vi "Measure_Main.vi"(0 "time target (s)":dbl, 1 "Upper limit of pH Value":dbl, 2 "Lower limit of pH Value":dbl, 3 "Upper limit of TEM":dbl, 4 "Lower limit of TEM":dbl, 8 "Upper limit of DO":dbl, 10 "Lower limit of DO":dbl) -> (7 "Maximum Alarm_pH":bool, 11 "Minumum Alarm_pH":bool, 14 "Voltage_pH":dbl, 15 "Maximum Alarm_TEM":bool, 16 "Minumum Alarm_TEM":bool, 17 "Maximum Alarm_DO":bool, 18 "Minumum Alarm_DO":bool)   [LabVIEW 2017]
uses:
  <vilib>/myRIO/Instrument Drivers/Onboard IO/AI/typedefs/AI Reference.ctl
  <vilib>/myRIO/Common/Instrument Driver Framework/Utilities/typedefs/myRIO Generic Hardware Reference.ctl
  <vilib>/myRIO/Common/Instrument Driver Framework/Utilities/typedefs/Hardware Version Enum.ctl
  <vilib>/myRIO/Common/Instrument Driver Framework/Utilities/typedefs/myRIO v1.0 Reference.ctl
  <vilib>/myRIO/Common/Instrument Driver Framework/Utilities/typedefs/Generic FPGA Reference.ctl
  <vilib>/myRIO/Common/Instrument Driver Framework/myRIO v1.0/AI/typedefs/AI Channels List.ctl
  <vilib>/myRIO/Common/Instrument Driver Framework/myRIO v1.0/AI/typedefs/AI Channels Enum.ctl
  <vilib>/myRIO/Common/Instrument Driver Framework/Utilities/typedefs/Analog Scaling Constants List.ctl
  <vilib>/myRIO/Common/Instrument Driver Framework/Utilities/typedefs/Analog Scaling Constants.ctl
  <vilib>/userdefined/High Color/nirio_resource_hc.ctl
  <vilib>/myRIO/Common/Instrument Driver Framework/myRIO v1.0/AI/vis/myRIO v1.1 Open AI.vi
  <vilib>/myRIO/Common/Instrument Driver Framework/Utilities/vis/Validate Channels.vi
  <vilib>/myRIO/Common/Instrument Driver Framework/myRIO v1.0/AI/vis/myRIO v1.0 Reserve AI.vi
  <vilib>/myRIO/Common/Instrument Driver Framework/myRIO v1.0/AI/vis/myRIO v1.0 Close AI.vi
  <vilib>/myRIO/Common/Instrument Driver Framework/myRIO v1.0/AI/vis/myRIO v1.0 Build MUX Configuration AI.vi
  <vilib>/myRIO/Common/Instrument Driver Framework/myRIO v1.0/Resource Manager/vis/myRIO v1.0 Reserve Channel List.vi
  <vilib>/myRIO/Common/Instrument Driver Framework/myRIO v1.0/AI/vis/myRIO v1.0 Unreserve AI.vi
  <vilib>/myRIO/Common/Instrument Driver Framework/myRIO v1.0/Resource Manager/vis/myRIO v1.0 Reserve Channel.vi
  <vilib>/myRIO/Common/Instrument Driver Framework/myRIO v1.0/Resource Manager/vis/myRIO v1.0 Unreserve Channel.vi
  <vilib>/myRIO/Common/Instrument Driver Framework/myRIO v1.0/Resource Manager/vis/myRIO v1.0 Unreserve Channel List.vi
  <vilib>/myRIO/Common/Instrument Driver Framework/myRIO v1.0/Resource Manager/vis/myRIO v1.0 Build Mutex Name.vi
  <vilib>/Utility/VariantDataType/GetNumericInfo.vi
  <vilib>/Utility/error.llb/Error Cluster From Error Code.vi
  <vilib>/myRIO/Common/Instrument Driver Framework/myRIO v1.0/myRIO v1.1 Open.vi
  <vilib>/myRIO/Common/Instrument Driver Framework/myRIO v1.0/AI/vis/myRIO v1.0 Get Scaling Constants AI.vi
  <vilib>/myRIO/Common/Instrument Driver Framework/Utilities/vis/IO Manager.vi
  <vilib>/myRIO/Common/Instrument Driver Framework/Utilities/vis/Configuration Manager.vi
  <vilib>/myRIO/Common/Instrument Driver Framework/myRIO v1.0/myRIO v1.0 Close.vi
  <vilib>/myRIO/Common/Instrument Driver Framework/myRIO v1.0/AI/vis/myRIO v1.0 Read AI.vi
  <vilib>/myRIO/Instrument Drivers/Onboard IO/AI/vis/myRIO AI Open.xnode
  <vilib>/myRIO/Instrument Drivers/Onboard IO/AI/AI.lvlib
panel:
  out "Voltage_Temperature":dbl
  out "Voltage_DO":dbl
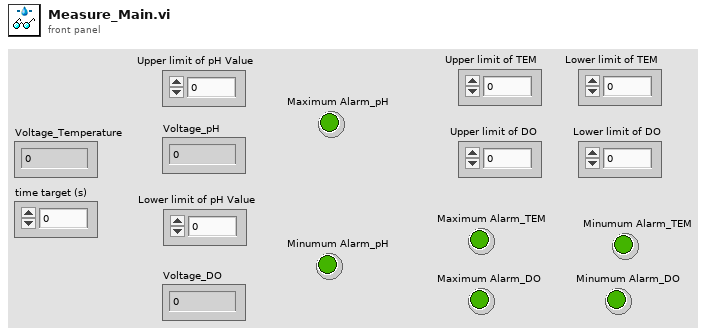
[diagram p1: front panel]
types:
  T1 = typedef "AI.lvlib/AI Reference.ctl" = cluster{"myRIO Reference":T2, "AI Channels List":T6, "AI Scaling Constants List":T8}
  T2 = typedef "myRIO Generic Hardware Reference.ctl" = cluster{"myRIO Model":T3, "myRIO Hardware Reference":T4}
  T3 = typedef "Hardware Version Enum.ctl" = enum16{"Unknown", "myRIO-1900", "myRIO-1950", "roboRIO", "NI ELVIS RIO CM"}
  T4 = typedef "myRIO v1.0 Reference.ctl" = cluster{"Generic FPGA Reference":T5, "Allow multiple opens":bool}
  T5 = typedef "Generic FPGA Reference.ctl" = refnum<k20>
  T6 = typedef "AI Channels List.ctl" = T7[]
  T7 = typedef "AI Channels Enum.ctl" = enum16{"Not Connected", "AudioIn/Left", "AudioIn/Right", "C/AI0", "C/AI1", "A/AI0", "A/AI1", "A/AI2", "A/AI3", "B/AI0", "B/AI1", "B/AI2", "B/AI3", "AI/AI0", "AI/AI1", "AI/AI2", "AI/AI3"}
  T8 = typedef "Analog Scaling Constants List.ctl" = T9[]
  T9 = typedef "Analog Scaling Constants.ctl" = cluster{"LSB Weight (Volts)":dbl, "Offset (Volts)":dbl, "Signed?":bool}
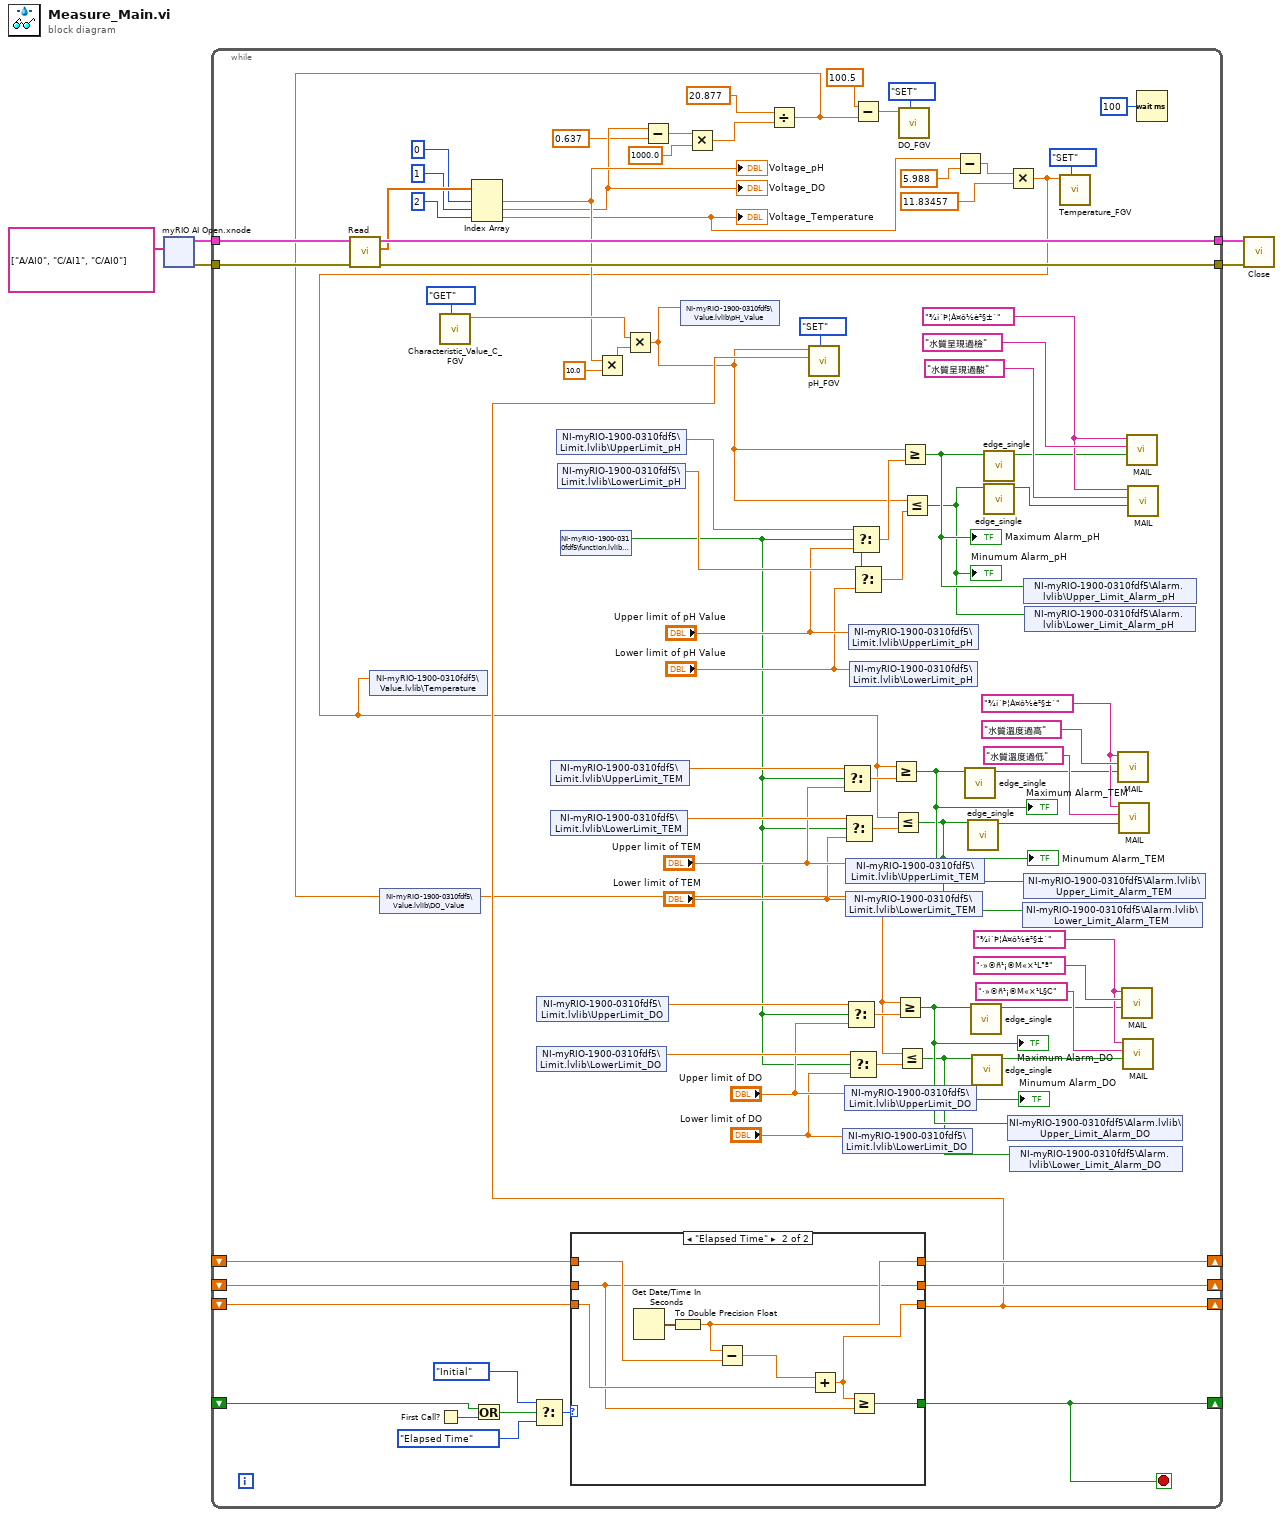
[diagram p0: block diagram]
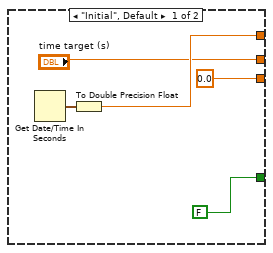
[diagram p2: hidden frame]
diagram:
  n1 = xnode "myRIO AI Open.xnode"("Channel Names"=tag[] ["A/AI0", "C/AI1", "C/AI0"]) -> ("error out"=w4:errorcluster, "AI Ref Out"=w5:T1)  [unwired: 2 in]
  n2 = while {
    tunnel: w5 -> [w80]
    tunnel: w4 -> [w79]
    tunnel: [w78] -> w3
    tunnel: [w77] -> w2
    shift-right: [w64] -> _
    shift-left: _ -> [w67]
    shift-right: [w63] -> _
    shift-left: _ -> [w66]
    shift-right: [w61] -> _
    shift-left: _ -> [w65]
    shift-right: [w6] -> _
    shift-left: _ -> [w62]
    stop <- w6 stop-if-true
    w39 = "¾i´Þ¦À¤ô½è²§±`" ("標題")
    w46 = "¾i´Þ¦À¤ô½è²§±`" ("標題")
    w84 = "¾i´Þ¦À¤ô½è²§±`" ("標題")
    n3 = call <vilib>:"Read.vi"("error in (no error)"=w79, "AI Ref In"=w80) -> ("error out"=w77:errorcluster, "Values"=w76:dbl[], "AI Ref Out"=w78:T1)  [unwired: 7 in]
    n4 = First Call?() -> (First Call?: T/F=w69:bool)
    n5 = call "Characteristic_Value_C_FGV.vi"("Command"=enum16{"SET", "GET"}."GET") -> ("Characteristic_Value_C_OUT"=w86:dbl)  [unwired: 9 in, 1 out]
    n6 = Index Array(array=w76, index #1=0 ("index"), index #2=1 ("index"), index #3=2 ("index")) -> (element #1=w74:dbl, element #2=w13:dbl, element #3=w59:dbl)
    "Voltage_pH" <- w74
    "Voltage_DO" <- w13
    "Voltage_Temperature" <- w59
    n7 = Or(x=w62, y=w69) -> (x .or. y?=w70:bool)
    n8 = Select(t=enum16{"Initial", "Elapsed Time"}."Initial", s=w70, f=enum16{"Initial", "Elapsed Time"}."Elapsed Time") -> (s? t:f=w71:enum16{"Initial", "Elapsed Time"})
    n9 = shared-variable "NI-myRIO-1900-0310fdf5\\Limit.lvlib\\UpperLimit_DO"() -> (w37:dbl)  [unwired: 1 in, 1 out]
    n10 = shared-variable "NI-myRIO-1900-0310fdf5\\Limit.lvlib\\LowerLimit_DO"() -> (w36:dbl)  [unwired: 1 in, 1 out]
    n11 = shared-variable "NI-myRIO-1900-0310fdf5\\Limit.lvlib\\UpperLimit_TEM"() -> (w44:dbl)  [unwired: 1 in, 1 out]
    n12 = shared-variable "NI-myRIO-1900-0310fdf5\\Limit.lvlib\\LowerLimit_TEM"() -> (w43:dbl)  [unwired: 1 in, 1 out]
    n13 = shared-variable "NI-myRIO-1900-0310fdf5\\Limit.lvlib\\UpperLimit_pH"() -> (w53:dbl)  [unwired: 1 in, 1 out]
    n14 = shared-variable "NI-myRIO-1900-0310fdf5\\Limit.lvlib\\LowerLimit_pH"() -> (w54:dbl)  [unwired: 1 in, 1 out]
    n15 = shared-variable "NI-myRIO-1900-0310fdf5\\function.lvlib\\Start"() -> (w30:bool)  [unwired: 1 in, 1 out]
    n16 = case shown="\"Elapsed Time\"" w71 {
      tunnel: ["time target (s)" w98] -> w63
      tunnel: w66 -> [_ w98]
      tunnel: [w93 w101] -> w64
      tunnel: w67 -> [_ w102]
      tunnel: [0.0 w97] -> w61
      tunnel: w65 -> [_ w100]
      tunnel: [FALSE w99] -> w6
      frame "Initial", Default {
        n17 = Get Date/Time In Seconds() -> (seconds since 1Jan1904=w94:timestamp)
        n18 = To Double Precision Float(number=w94) -> (double precision float=w93:dbl)
      }
      frame "Elapsed Time" {
        n19 = Get Date/Time In Seconds() -> (seconds since 1Jan1904=w103:timestamp)
        n20 = To Double Precision Float(number=w103) -> (double precision float=w101:dbl)
        n21 = Subtract(x=w101, y=w102) -> (x-y=w96:dbl)
        n22 = Add(x=w96, y=w100) -> (x+y=w97:dbl)
        n23 = Greater Or Equal?(x=w97, y=w98) -> (x >= y?=w99:bool)
      }
    }
    n24 = Multiply(x=w74, y=10.0) -> (x*y=w87:dbl)
    n25 = Multiply(x=w86, y=w87) -> (x*y=w52:dbl)
    n26 = Subtract(x=w13, y=0.637) -> (x-y=w11:dbl)
    n27 = shared-variable "NI-myRIO-1900-0310fdf5\\Value.lvlib\\pH_Value"(w52) -> ()  [unwired: 1 in, 1 out]
    n28 = Multiply(x=w11, y=1000.0) -> (x*y=w10:dbl)
    n29 = Divide(x=20.877, y=w10) -> (x/y=w8:dbl)
    n30 = shared-variable "NI-myRIO-1900-0310fdf5\\Value.lvlib\\DO_Value"(w8) -> ()  [unwired: 1 in, 1 out]
    n31 = call "pH_FGV.vi"("Command"=enum16{"SET", "GET"}."SET", "Elapsed_Time(s)"=w61, "pH_Value_IN"=w52) -> ()  [unwired: 6 in, 3 out]
    n32 = Select(t=w44, s=w30, f="Upper limit of TEM") -> (s? t:f=w49:dbl)
    n33 = shared-variable "NI-myRIO-1900-0310fdf5\\Limit.lvlib\\LowerLimit_DO"("Lower limit of DO") -> ()  [unwired: 1 in, 1 out]
    n34 = Select(t=w43, s=w30, f="Lower limit of TEM") -> (s? t:f=w48:dbl)
    n35 = shared-variable "NI-myRIO-1900-0310fdf5\\Limit.lvlib\\UpperLimit_DO"("Upper limit of DO") -> ()  [unwired: 1 in, 1 out]
    n36 = shared-variable "NI-myRIO-1900-0310fdf5\\Limit.lvlib\\UpperLimit_TEM"("Upper limit of TEM") -> ()  [unwired: 1 in, 1 out]
    n37 = shared-variable "NI-myRIO-1900-0310fdf5\\Limit.lvlib\\LowerLimit_TEM"("Lower limit of TEM") -> ()  [unwired: 1 in, 1 out]
    n38 = Select(t=w37, s=w30, f="Upper limit of DO") -> (s? t:f=w42:dbl)
    n39 = Select(t=w36, s=w30, f="Lower limit of DO") -> (s? t:f=w41:dbl)
    n40 = shared-variable "NI-myRIO-1900-0310fdf5\\Limit.lvlib\\UpperLimit_pH"("Upper limit of pH Value") -> ()  [unwired: 1 in, 1 out]
    n41 = shared-variable "NI-myRIO-1900-0310fdf5\\Limit.lvlib\\LowerLimit_pH"("Lower limit of pH Value") -> ()  [unwired: 1 in, 1 out]
    n42 = Select(t=w53, s=w30, f="Upper limit of pH Value") -> (s? t:f=w89:dbl)
    n43 = Subtract(x=100.5, y=w8) -> (x-y=w9:dbl)
    n44 = Select(t=w54, s=w30, f="Lower limit of pH Value") -> (s? t:f=w88:dbl)
    n45 = Greater Or Equal?(x=w8, y=w42) -> (x >= y?=w18:bool)
    "Maximum Alarm_DO" <- w18
    n46 = Less Or Equal?(x=w8, y=w41) -> (x <= y?=w16:bool)
    "Minumum Alarm_DO" <- w16
    n47 = call "DO_FGV.vi"("Command"=enum16{"SET", "GET"}."SET", "DO_Value_IN"=w9) -> ()  [unwired: 8 in, 2 out]
    n48 = Greater Or Equal?(x=w52, y=w89) -> (x >= y?=w26:bool)
    "Maximum Alarm_pH" <- w26
    n49 = Less Or Equal?(x=w52, y=w88) -> (x <= y?=w24:bool)
    "Minumum Alarm_pH" <- w24
    n50 = Subtract(x=w59, y=5.988) -> (x-y=w58:dbl)
    n51 = call "edge_single.vi"("DI Value"=w18) -> ("DO Value"=w17:bool)  [unwired: 10 in]
    n52 = call "edge_single.vi"("DI Value"=w16) -> ("DO Value"=w15:bool)  [unwired: 10 in]
    n53 = call "edge_single.vi"("DI Value"=w26) -> ("DO Value"=w25:bool)  [unwired: 10 in]
    n54 = call "edge_single.vi"("DI Value"=w24) -> ("DO Value"=w23:bool)  [unwired: 10 in]
    n55 = Multiply(x=w58, y=11.83457) -> (x*y=w35:dbl)
    n56 = shared-variable "NI-myRIO-1900-0310fdf5\\Value.lvlib\\Temperature"(w35) -> ()  [unwired: 1 in, 1 out]
    n57 = Greater Or Equal?(x=w35, y=w49) -> (x >= y?=w22:bool)
    "Maximum Alarm_TEM" <- w22
    n58 = Less Or Equal?(x=w35, y=w48) -> (x <= y?=w20:bool)
    "Minumum Alarm_TEM" <- w20
    n59 = call "edge_single.vi"("DI Value"=w22) -> ("DO Value"=w21:bool)  [unwired: 10 in]
    n60 = call "edge_single.vi"("DI Value"=w20) -> ("DO Value"=w19:bool)  [unwired: 10 in]
    n61 = shared-variable "NI-myRIO-1900-0310fdf5\\Alarm.lvlib\\Upper_Limit_Alarm_DO"(w18) -> ()  [unwired: 1 in, 1 out]
    n62 = shared-variable "NI-myRIO-1900-0310fdf5\\Alarm.lvlib\\Lower_Limit_Alarm_DO"(w16) -> ()  [unwired: 1 in, 1 out]
    n63 = shared-variable "NI-myRIO-1900-0310fdf5\\Alarm.lvlib\\Lower_Limit_Alarm_TEM"(w20) -> ()  [unwired: 1 in, 1 out]
    n64 = shared-variable "NI-myRIO-1900-0310fdf5\\Alarm.lvlib\\Upper_Limit_Alarm_pH"(w26) -> ()  [unwired: 1 in, 1 out]
    n65 = shared-variable "NI-myRIO-1900-0310fdf5\\Alarm.lvlib\\Upper_Limit_Alarm_TEM"(w22) -> ()  [unwired: 1 in, 1 out]
    n66 = shared-variable "NI-myRIO-1900-0310fdf5\\Alarm.lvlib\\Lower_Limit_Alarm_pH"(w24) -> ()  [unwired: 1 in, 1 out]
    n67 = call "Temperature_FGV.vi"("Command"=enum16{"SET", "GET"}."SET", "Temperature_IN"=w35) -> ()  [unwired: 8 in, 2 out]
    n68 = call "MAIL.vi"("±H°e"=w21, "內容"="水質溫度過高", "標題"=w46) -> ()  [unwired: 9 in]
    n69 = call "MAIL.vi"("±H°e"=w19, "內容"="水質溫度過低", "標題"=w46) -> ()  [unwired: 9 in]
    n70 = call "MAIL.vi"("±H°e"=w17, "內容"="·»®ñ¹¡©M«×¹L°ª", "標題"=w39) -> ()  [unwired: 9 in]
    n71 = call "MAIL.vi"("±H°e"=w15, "內容"="·»®ñ¹¡©M«×¹L§C", "標題"=w39) -> ()  [unwired: 9 in]
    n72 = call "MAIL.vi"("±H°e"=w25, "內容"="水質呈現過檢", "標題"=w84) -> ()  [unwired: 9 in]
    n73 = call "MAIL.vi"("±H°e"=w23, "內容"="水質呈現過酸", "標題"=w84) -> ()  [unwired: 9 in]
    n74 = Wait (ms)(milliseconds to wait=u32 100) -> ()  [unwired: 1 out]
  }
  n75 = call <vilib>:"Close.vi"("error in (no error)"=w2, "AI Ref In"=w3) -> ()  [unwired: 9 in, 1 out]
